vi "StopDAQmxTasks.vi"(8 "error in (no error)":errorcluster caption="entrée d'erreur (pas d'erreur)", 11 "Control en entrée":refnum<class "Control-Server.lvclass">) -> (0 "error out":errorcluster caption="sortie d'erreur", 3 "Control en sortie":refnum<class "Control-Server.lvclass">)   [LabVIEW 2015, in "Control-Server.lvclass"]
uses:
  Control-Server.lvclass
  Config/config_names_def.ctl
  Config/Config.lvclass/Config.ctl
  DAQmxTasks/DAQmxTask.lvclass
  Config/Config.lvclass
  DAQmxTasks/DAQmxTaskContainer_General/DAQmxTaksContainer_General.lvclass
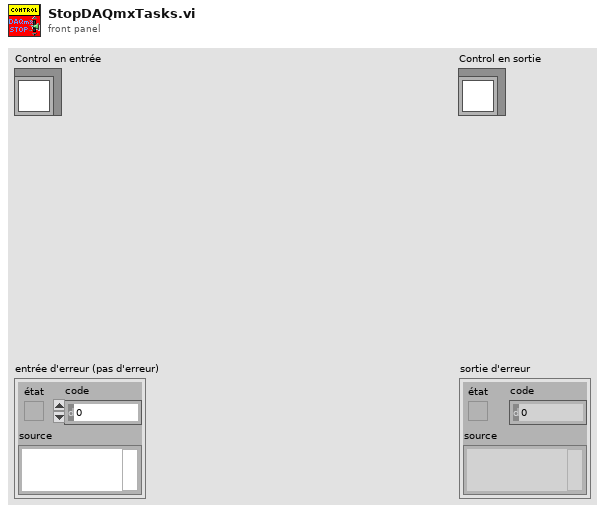
[diagram p1: front panel]
types:
  T1 = typedef "Config.lvclass/config_names_def.ctl" = string
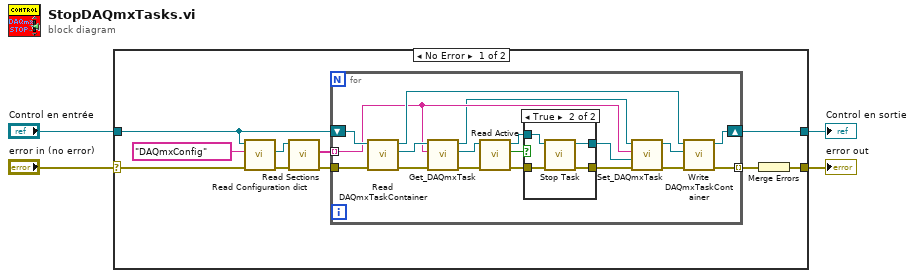
[diagram p0: block diagram]
diagram:
  n1 = case shown="No Error" "error in (no error)" {
    selector: "error in (no error)" -> [w12 w40]
    tunnel: [w13 w40] -> w3
    tunnel: [w14 w39] -> w1
    tunnel: "Control en entrée" -> [w5 w39]
    frame No Error {
      n2 = call "Read Configuration dict.vi"("error in (no error)"=w12, "Config Name"=T1 "DAQmxConfig", "Control in"=w5) -> ("error out"=w9:errorcluster, "Config"=w11:refnum<class "Config.lvclass">)  [unwired: 6 in, 1 out]
      n3 = call "Read Sections.vi"("error in (no error)"=w9, "Config in"=w11) -> ("error out"=w7:errorcluster, "Sections"=w8:string[])  [unwired: 7 in, 1 out]
      n4 = for {
        tunnel: w8 -> [w21] mode=indexing
        shift-right: [w25] -> w14
        shift-left: w5 -> [w29]
        tunnel: w7 -> [w28]
        tunnel: [w18] -> w6 mode=indexing
        n5 = call-dynamic "Read DAQmxTaskContainer.vi"("error in (no error)"=w28, "Control in"=w29) -> ("error out"=w26:errorcluster, "DAQmxTaksContainer_General.lvclass"=w27:refnum<class "DAQmxTaksContainer_General.lvclass">, "Control out"=w24:refnum<class "Control-Server.lvclass">)  [unwired: 7 in]
        n6 = call "Get_DAQmxTask.vi"("error in (no error)"=w26, "Task name"=w21, "DAQmxTaksContainer_General in"=w27) -> ("error out"=w16:errorcluster, "DAQmx Task"=w17:refnum<class "DAQmxTask.lvclass">, "DAQmxTaksContainer_General out"=w20:refnum<class "DAQmxTaksContainer_General.lvclass">)  [unwired: 6 in]
        n7 = call-dynamic "Read Active.vi"("error in (no error)"=w16, "DAQmxTask in"=w17) -> ("error out"=w32:errorcluster, "Active?"=w31:bool, "DAQmxTask out"=w30:refnum<class "DAQmxTask.lvclass">)  [unwired: 7 in]
        n8 = case shown="True" w31 {
          tunnel: [w33 w38] -> w19
          tunnel: w30 -> [w34 w37]
          tunnel: w32 -> [w33 w36]
          tunnel: [w34 w35] -> w15
          frame False {
          }
          frame True {
            n9 = call "Stop Task.vi"("error in (no error)"=w36, "DAQmxTask in"=w37) -> ("error out"=w38:errorcluster, "DAQmxTask out"=w35:refnum<class "DAQmxTask.lvclass">)  [unwired: 8 in]
          }
        }
        n10 = call "Set_DAQmxTask.vi"("error in (no error)"=w19, "DAQmxTask"=w15, "Task name"=w21, "DAQmxTaksContainer_General in"=w20) -> ("error out"=w22:errorcluster, "DAQmxTaksContainer_General out"=w23:refnum<class "DAQmxTaksContainer_General.lvclass">)  [unwired: 6 in]
        n11 = call-dynamic "Write DAQmxTaskContainer.vi"("error in (no error)"=w22, "DAQmxTaksContainer_General.lvclass"=w23, "Control in"=w24) -> ("error out"=w18:errorcluster, "Control out"=w25:refnum<class "Control-Server.lvclass">)  [unwired: 7 in]
      }
      n12 = Merge Errors(w6) -> (w13:errorcluster)
    }
    frame Error {
    }
  }
  "error out" <- w3
  "Control en sortie" <- w1
